vi "Get TimeStamp Formatted.vi"(8 "error in (no error)":errorcluster, 11 "Interface_Class in":refnum<class "Abstraction_Interface_Class.lvclass">) -> (0 "error out":errorcluster, 1 "TimeStamp Formatted":string, 3 "Interface_Class out":refnum<class "Abstraction_Interface_Class.lvclass">)   [LabVIEW 2023, in "Abstraction_Interface.lvlib" / "Abstraction_Interface_Class.lvclass"]
uses:
  Abstraction_Interface_Class.lvclass
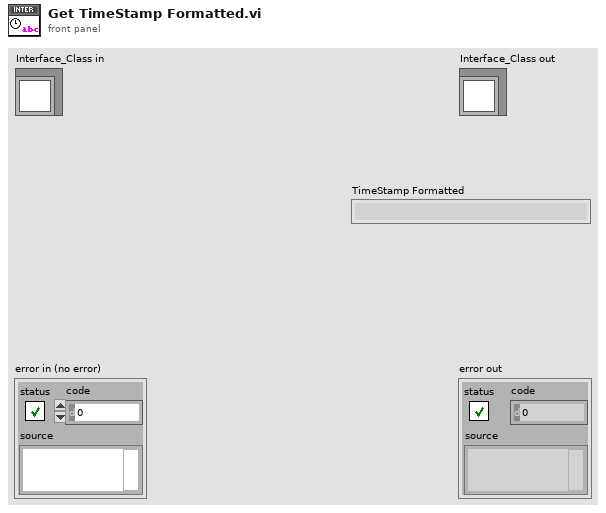
[diagram p1: front panel]
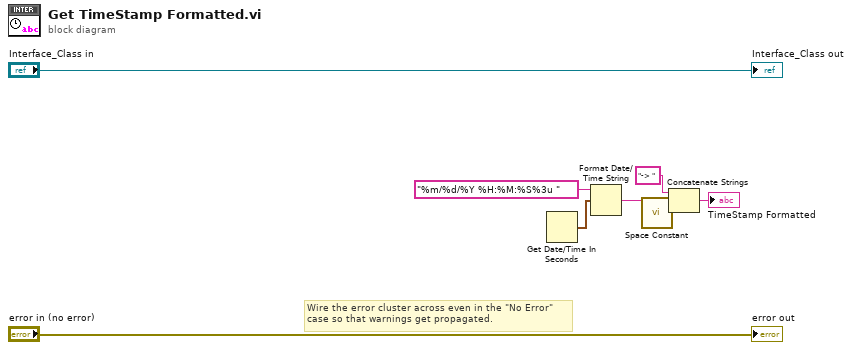
[diagram p0: block diagram]
diagram:
  # "Wire the error cluster across even in the \"No Error\"\ncase so that warnings get propagated."
  n1 = Get Date/Time In Seconds() -> (seconds since 1Jan1904=w6:timestamp)
  n2 = Format Date/Time String(time format string (%c)="%m/%d/%Y %H:%M:%S%3u " ("format string"), seconds (now)=w6) -> (date/time string=w4:string)  [unwired: 1 in]
  n3 = call <vilib>:"Space Constant.vi"() -> ("String"=w2:string)
  n4 = Concatenate Strings("-> " ("string"), w4, w2) -> (→"TimeStamp Formatted":string)
  "error out" <- "error in (no error)"
  "Interface_Class out" <- "Interface_Class in"
